vi "Stepper construct.vi"() -> ()   [LabVIEW 2015]
uses:
  <vilib>/LabVIEW Targets/FPGA/cRIO/shared/nicrio_ModuleControls/nicrio_cRIO-950x_DriveStatus.ctl
  <vilib>/LabVIEW Targets/FPGA/cRIO/shared/nicrio_ModuleControls/nicrio_cRIO-9501_MicrostepRate.ctl
  <vilib>/LabVIEW Targets/FPGA/cRIO/shared/nicrio_ModuleControls/nicrio_cRIO-9501_CurrentReducPer.ctl
panel:
  in  "x":dbl=-4000.0 format="%#_13g"
  in  "Manual":bool
  in  "Reset":bool
  out "Waveform Chart 4":dbl(graph)
  out "Waveform Chart 3":cluster{"Double":dbl, "Setpoint (1)":dbl}(graph)
  out "In Range?":bool
  out "Output":dbl=0.01
  in  "PID":cluster{"P":dbl, "I":dbl, "D":dbl}={"P"=15.0, "I"=0.03000000000000002, "D"=0.30000000000000004}
  in  "Setpoint (1)":dbl=1.0 format="%.2g"
  in  "Vertical Pointer Slide":dbl(slide) scale=1.0..-1.0
  in  "Current Reduction Delay":u16
  in  "Current Reduction Percentage":T1
  in  "Rated Phase Current":fxp<+/-,12,4>=0.3984375 format="%#_10g"
  in  "Microstepping Rate":T2
  in  "Apply Configuration":bool
  out "Drive Status":T3
  in  "Enable Drive":bool
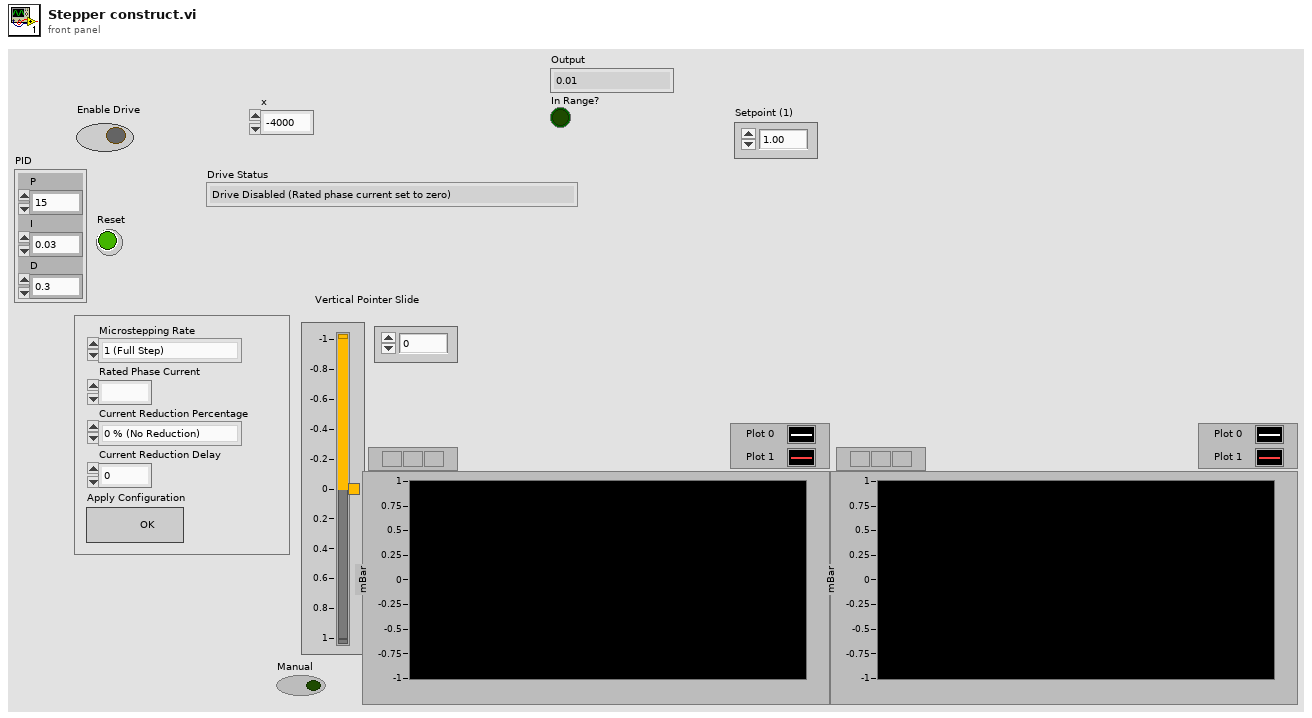
[diagram p1: front panel]
types:
  T1 = typedef "nicrio_cRIO-9501_CurrentReducPer.ctl" = enum8{"0 % (No Reduction)", "25 %", "50 %"}
  T2 = typedef "nicrio_cRIO-9501_MicrostepRate.ctl" = enum8{"1 (Full Step)", "2 (Half Step)", "4", "8", "16", "32", "64", "128", "256"}
  T3 = typedef "nicrio_cRIO-950x_DriveStatus.ctl" = enum8{"Drive Disabled (Rated phase current set to zero)", "Drive Disabled (Disabled by fault)", "Drive Disabled (Disabled by software)", "Drive Enabled"}
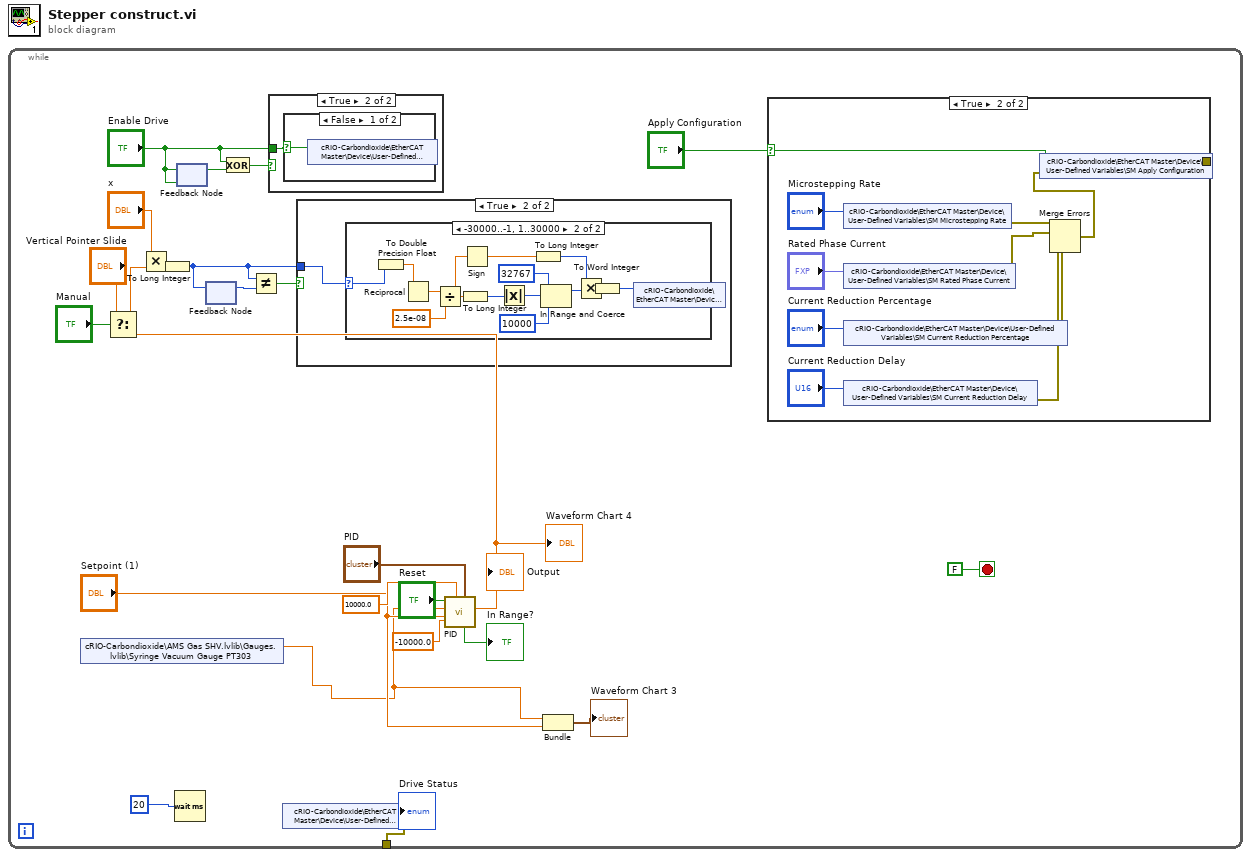
[diagram p0: block diagram]
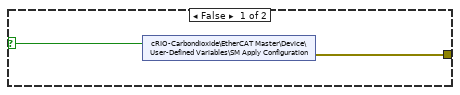
[diagram p2: hidden frame]
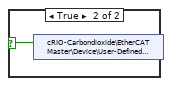
[diagram p6: hidden frame]
diagram:
  n1 = while {
    tunnel: [w16] -> _
    stop <- FALSE stop-if-true
    n2 = shared-variable "cRIO-Carbondioxide\\AMS Gas SHV.lvlib\\Gauges.lvlib\\Syringe Vacuum Gauge PT303"() -> (w6:dbl)  [unwired: 1 in, 1 out]
    n3 = Wait (ms)(milliseconds to wait=u32 20) -> ()  [unwired: 1 out]
    n4 = feedback #1("Enable Drive") -> (w23:bool)
    n5 = feedback-in #1("Enable Drive") -> ()
    n6 = feedback #2() -> (w21:i32)  [unwired: 1 in]
    n7 = Exclusive Or(1:w23, 2:"Enable Drive") -> (0:w24:bool)
    n8 = case shown="True" w24 {
      tunnel: "Enable Drive" -> [_ w54]
      frame False {
      }
      frame True {
        n9 = case shown="False" w54 {
          selector: w54 -> [w55 w56]
          frame False {
            n10 = shared-variable "cRIO-Carbondioxide\\EtherCAT Master\\Device\\User-Defined Variables\\SM Enable Drive"(w55) -> ()  [unwired: 1 in, 1 out]
          }
          frame True {
            n11 = shared-variable "cRIO-Carbondioxide\\EtherCAT Master\\Device\\User-Defined Variables\\SM Enable Drive"(w56) -> ()  [unwired: 1 in, 1 out]
          }
        }
      }
    }
    n12 = shared-variable "cRIO-Carbondioxide\\EtherCAT Master\\Device\\User-Defined Variables\\SM Drive Status"() -> (→"Drive Status":u8, error out=w16:errorcluster)  [unwired: 1 in]
    n13 = call "PID.vi"("PID"="PID", "Lower Limit"=-10000.0, "Upper Limit (0,01)"=10000.0, "Setpoint (0,002)"="Setpoint (1)", "Process"=w6, "Reset"="Reset") -> ("Output"=w1:dbl, "In Range?"=→"In Range?":bool)  [unwired: 4 in]
    "Output" <- w1
    "Waveform Chart 4" <- w1
    n14 = Select(t="Vertical Pointer Slide", s="Manual", f=w1) -> (s? t:f=w2:dbl)
    n15 = Multiply(x="x", y=w2) -> (x*y=w10:dbl)
    n16 = To Long Integer(number=w10) -> (32bit integer=w8:i32)
    n17 = feedback-in #2(w8) -> ()
    n18 = Not Equal?(x=w8, y=w21) -> (x != y?=w20:bool)
    n19 = case shown="True" w20 {
      tunnel: w8 -> [_ w39]
      frame False {
      }
      frame True {
        n20 = case shown="-30000..-1, 1..30000" w39 {
          selector: w39 -> [_ w49]
          frame 0, Default {
          }
          frame -30000..-1, 1..30000 {
            n21 = To Double Precision Float(number=w49) -> (double precision float=w53:dbl)
            n22 = Reciprocal(x=w53) -> (1/x=w52:dbl)
            n23 = Divide(x=w52, y=2.5e-08) -> (x/y=w50:dbl)
            n24 = To Long Integer(number=w50) -> (32bit integer=w48:i32)
            n25 = Sign(1:w50) -> (0:w44:dbl)
            n26 = Absolute Value(x=w48) -> (abs(x)=w47:i32)
            n27 = To Long Integer(number=w44) -> (32bit integer=w43:i32)
            n28 = In Range and Coerce(upper limit=32767, x=w47, lower limit=10000) -> (coerced(x)=w45:i32)  [unwired: 1 out]
            n29 = Multiply(x=w43, y=w45) -> (x*y=w42:i32)
            n30 = To Word Integer(number=w42) -> (16bit integer=w40:i16)
            n31 = shared-variable "cRIO-Carbondioxide\\EtherCAT Master\\Device\\User-Defined Variables\\SM Ticks"(w40) -> ()  [unwired: 1 in, 1 out]
          }
        }
      }
    }
    n32 = Bundle("Double"=w6, "Setpoint (1)"="Setpoint (1)") -> (→"Waveform Chart 3":cluster{"Double":dbl, "Setpoint (1)":dbl})  [unwired: 1 in]
    n33 = case shown="True" "Apply Configuration" {
      selector: "Apply Configuration" -> [w27 w30]
      tunnel: [w26 w28] -> _
      frame False {
        n34 = shared-variable "cRIO-Carbondioxide\\EtherCAT Master\\Device\\User-Defined Variables\\SM Apply Configuration"(w27) -> (error out=w26:errorcluster)  [unwired: 1 in]
      }
      frame True {
        n35 = shared-variable "cRIO-Carbondioxide\\EtherCAT Master\\Device\\User-Defined Variables\\SM Microstepping Rate"("Microstepping Rate") -> (error out=w34:errorcluster)  [unwired: 1 in]
        n36 = shared-variable "cRIO-Carbondioxide\\EtherCAT Master\\Device\\User-Defined Variables\\SM Rated Phase Current"("Rated Phase Current") -> (error out=w33:errorcluster)  [unwired: 1 in]
        n37 = shared-variable "cRIO-Carbondioxide\\EtherCAT Master\\Device\\User-Defined Variables\\SM Current Reduction Percentage"("Current Reduction Percentage") -> (error out=w32:errorcluster)  [unwired: 1 in]
        n38 = shared-variable "cRIO-Carbondioxide\\EtherCAT Master\\Device\\User-Defined Variables\\SM Current Reduction Delay"("Current Reduction Delay") -> (error out=w31:errorcluster)  [unwired: 1 in]
        n39 = Merge Errors(w34, w33, w32, w31) -> (w29:errorcluster)
        n40 = shared-variable "cRIO-Carbondioxide\\EtherCAT Master\\Device\\User-Defined Variables\\SM Apply Configuration"(w30, error in=w29) -> (error out=w28:errorcluster)
      }
    }
  }
